vi "Compile VR-Hall.vi"(8 "error in (no error)":errorcluster, 10 "PB-01 Compiled Data":T1, 11 "Device Item Ref in":T4 format="%.0x") -> (0 "error out":errorcluster, 2 "PB-01 Compiled Data out":T1, 3 "Device Item Ref out":T4 format="%.0x")   [LabVIEW 2015, in "DCM System Explorer.lvlib"]
uses:
  DCM System Explorer.lvlib
  <vilib>/NI Veristand/Custom Device API/Custom Device Item Ref.ctl
  Shared/Types/PB-01.ctl
  Shared/Types/ESTTL Setup Indexes.ctl
  <vilib>/Powertrain Controls/Device Drivers/VR-Hall/RevC/Real-Time/Support/Vr_Hall_mode_control_revc.ctl
  Shared/DCM Properties.vi
  Shared/DCM Constants and GUIDs.vi
  <vilib>/NI Veristand/Custom Device Tools/Custom Device Utility Library/NI VeriStand - Search for Item by GUID.vi
  <vilib>/NI Veristand/Custom Device API/Get Item Property (Double Array).vi
  <vilib>/NI Veristand/Custom Device Tools/Custom Device Utility Library/Custom Device Utility Library.lvlib
  <vilib>/NI VeriStand/Custom Device API/Custom Device API.lvlib
  DCM Shared.lvlib
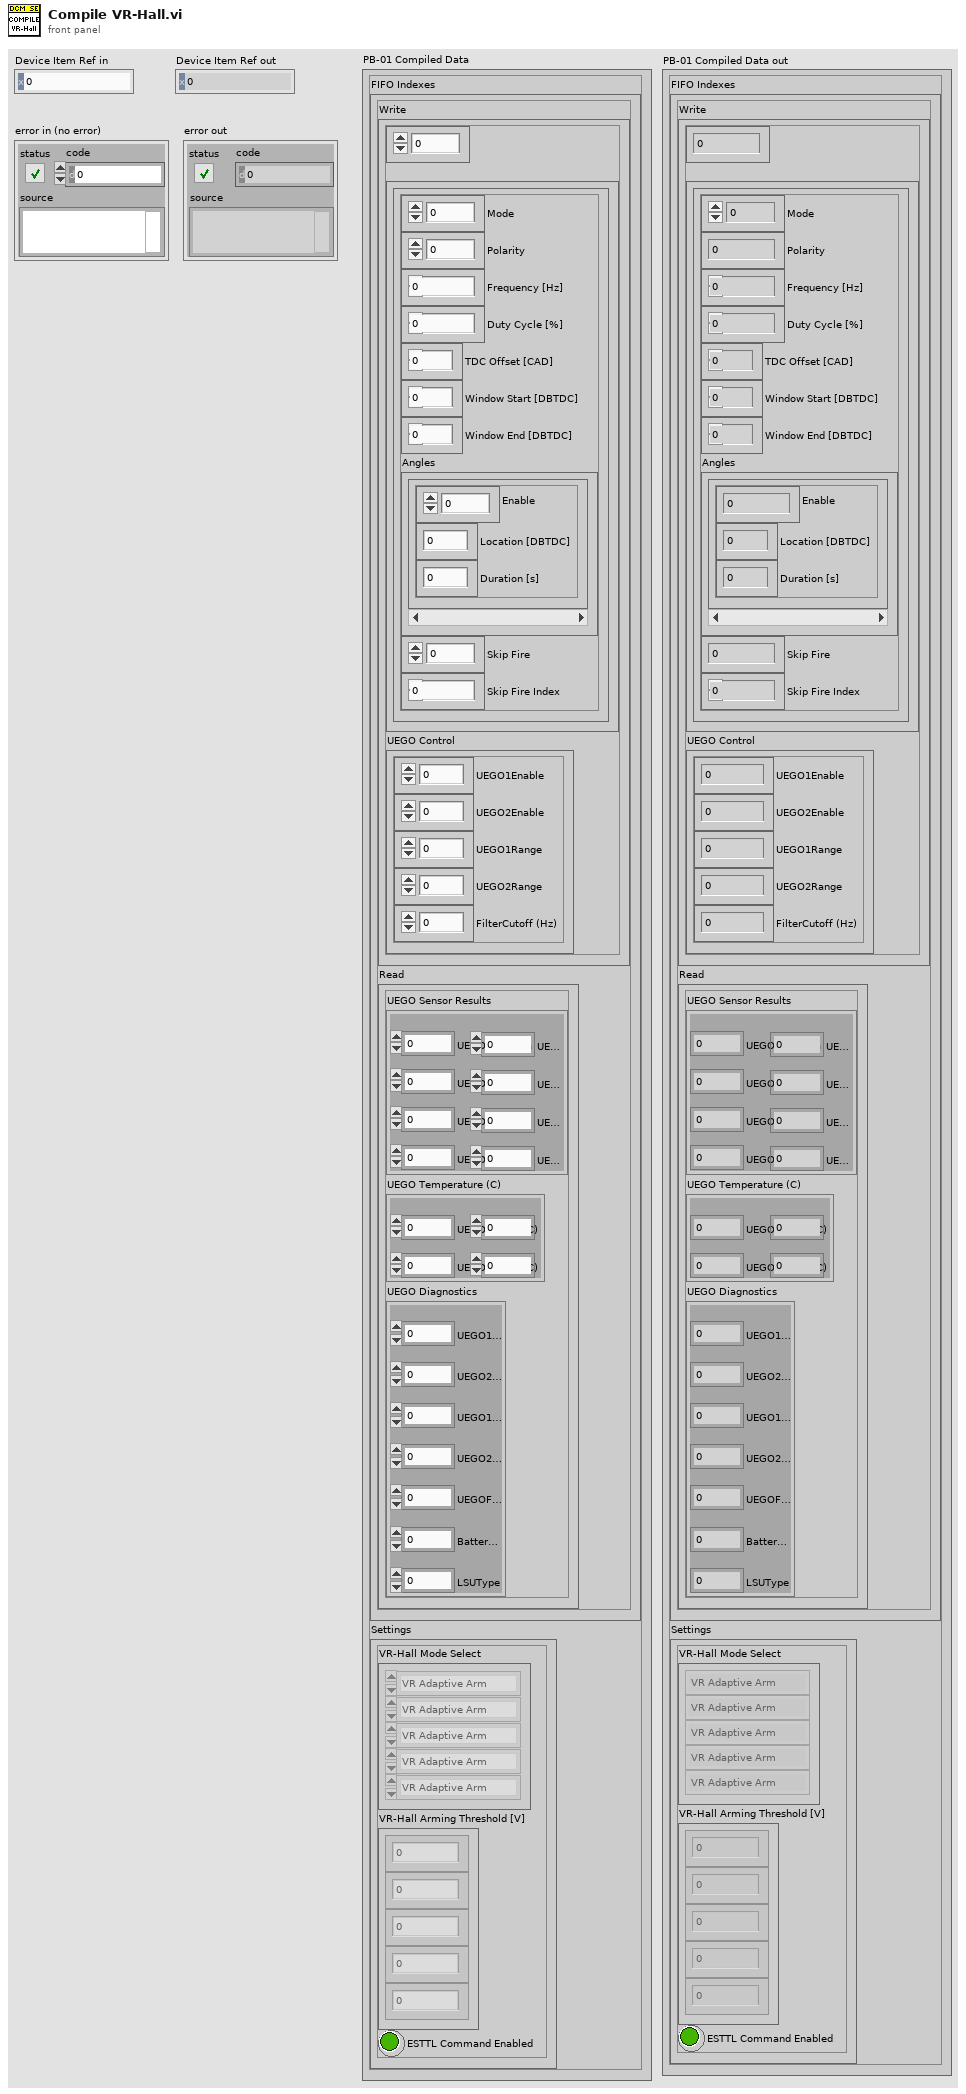
[diagram p1: front panel]
types:
  T1 = typedef "DCM Shared.lvlib/PB-01.ctl" = cluster{"FIFO Indexes":cluster{"Write":cluster{"Clear Faults":i32, "ESTTL Setup":T2[], "UEGO Control":cluster{"UEGO1Enable":i32, "UEGO2Enable":i32, "UEGO1Range":i32, "UEGO2Range":i32, "FilterCutoff (Hz)":i32}}, "Read":cluster{"UEGO Sensor Results":cluster{"UEGO1Lambda":i32, "UEGO1Phi":i32, "UEGO1AFRatio":i32, "UEGO1Ip (mA)":i32, "UEGO2Lambda":i32, "UEGO2Phi":i32, "UEGO2AFRatio":i32, "UEGO2Ip (mA)":i32}, "UEGO Temperature (C)":cluster{"UEGO1Temp (C)":i32, "UEGO2Temp (C)":i32, "UEGO1Hot":i32, "UEGO2Hot":i32}, "UEGO Diagnostics":cluster{"UEGO1SensorFault":i32, "UEGO2SensorFault":i32, "UEGO1HeaterFault":i32, "UEGO2HeaterFault":i32, "UEGOFuseStatus":i32, "Battery (V)":i32, "LSUType":i32}}}, "Settings":cluster{"VR-Hall Mode Select":T3[], "VR-Hall Arming Threshold [V]":dbl[], "ESTTL Command Enabled":bool}}
  T2 = typedef "DCM Shared.lvlib/ESTTL Setup Indexes.ctl" = cluster{"Mode":i32, "Polarity":i32, "Frequency [Hz]":i32, "Duty Cycle [%]":i32, "TDC Offset [CAD]":i32, "Window Start [DBTDC]":i32, "Window End [DBTDC]":i32, "Angles":cluster{"Enable":i32, "Location [DBTDC]":i32, "Duration [s]":i32}[], "Skip Fire":i32, "Skip Fire Index":i32}
  T3 = typedef "Vr_Hall_mode_control_revc.ctl" = enum32{"VR Adaptive Arm", "VR Manual Arm", "Hall", "Hall w/ Pull-up"}
  T4 = typedef "Custom Device API.lvlib/Custom Device Item Ref.ctl" = u64
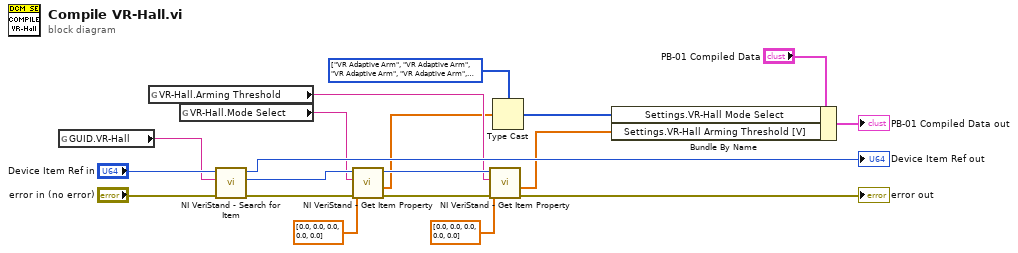
[diagram p0: block diagram]
diagram:
  w2 = T3[] [enum."VR Adaptive Arm", enum."VR Adaptive Arm", enum."VR Adaptive Arm", enum."VR Adaptive Arm", enum."VR Adaptive Arm"] items=["VR Adaptive Arm", "VR Manual Arm", "Hall", "Hall w/ Pull-up"] ("Settings.VR-Hall Mode Select")
  n1 = global read "DCM Constants and GUIDs.vi" "GUID.VR-Hall"() -> (w17:string)
  n2 = global read "DCM Properties.vi" "VR-Hall.Arming Threshold"() -> (w9:string)
  n3 = global read "DCM Properties.vi" "VR-Hall.Mode Select"() -> (w8:string)
  n4 = call-poly <vilib>:"NI VeriStand - Search for Item.vi"("error in"="error in (no error)", "Item GUID"=w17, "Section Ref in"="Device Item Ref in") -> ("error out"=w4:errorcluster, "Item Ref"=w10:T4, "Section Ref out"=→"Device Item Ref out":T4)  [unwired: 5 in, 1 out]
  n5 = call-poly <vilib>:"NI VeriStand - Get Item Property.vi"("error in (no error)"=w4, "Default Value"=dbl[] [0.0, 0.0, 0.0, 0.0, 0.0], "Property Name"=w8, "Item Ref in"=w10) -> ("error out"=w15:errorcluster, "Value"=w3:dbl[], "Item Ref out"=w13:T4)  [unwired: 4 in, 1 out]
  n6 = call-poly <vilib>:"NI VeriStand - Get Item Property.vi"("error in (no error)"=w15, "Default Value"=dbl[] [0.0, 0.0, 0.0, 0.0, 0.0], "Property Name"=w9, "Item Ref in"=w13) -> ("error out"=→"error out":errorcluster, "Value"=w7:dbl[])  [unwired: 4 in, 2 out]
  n7 = Type Cast(type=w2, x=w3) -> (*(type *) &x=w1:T3[])
  n8 = Bundle By Name(cluster="PB-01 Compiled Data", "Settings.VR-Hall Mode Select"=w1, "Settings.VR-Hall Arming Threshold [V]"=w7) -> (→"PB-01 Compiled Data out":T1)
